vi "Execute.vi"(0 "object in":refnum<class "IDataMethod.lvclass">, 2 "Requirements":T1={"From"=enum."TDMS", "File Handler"=variant, "Input"=variant(map{string, dbl[]} {})}, 5 "Error In":errorcluster) -> (14 "object out":refnum<class "IDataMethod.lvclass">, 16 "Message":T3, 19 "Error Out":errorcluster)   [LabVIEW 2024, in "IDataMethod.lvclass"]
doc: "Abstact execute method which represents either logging or viewing method."
uses:
  IDataMethod.lvclass
  Support/Type Def/Message.ctl
  Support/Type Def/Requirements.ctl
  Support/Type Def/File Type.ctl
panel:
  # "Connector Pane"
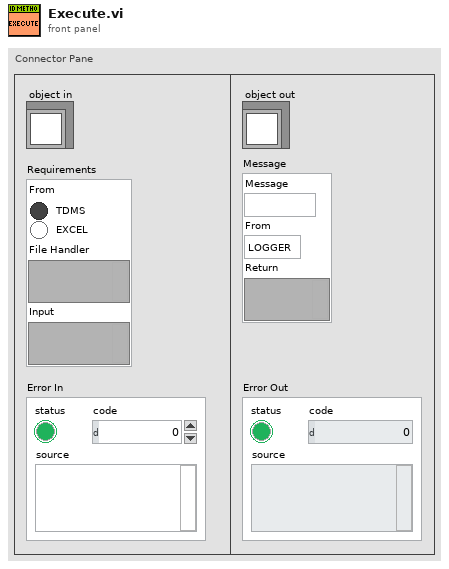
[diagram p1: front panel]
types:
  T1 = typedef "Requirements.ctl" = cluster{"From":T2, "File Handler":variant, "Input":variant}
  T2 = typedef "File Type.ctl" = enum32{"TDMS", "EXCEL"}
  T3 = typedef "Message.ctl" = cluster{"Message":string, "From":enum16{"LOGGER", "VIEWER"}, "Return":variant}
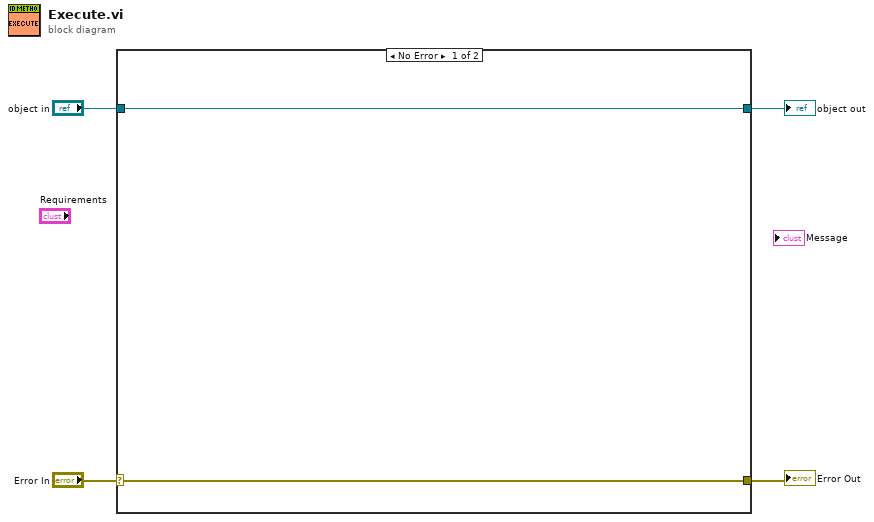
[diagram p0: block diagram]
diagram:
  n1 = case shown="No Error" "Error In" {
    selector: "Error In" -> [w6 w8]
    tunnel: [w6 w8] -> w3
    tunnel: [w5 w7] -> w1
    tunnel: "object in" -> [w5 w7]
    frame No Error {
    }
    frame Error {
    }
  }
  "Error Out" <- w3
  "object out" <- w1
